vi "AO Regs Group UI.vi"(8 "error in (no error)":errorcluster, 11 "Node Ptr":T2 format="%.0x") -> (0 "error out":errorcluster)   [LabVIEW 2015, in "Modbus Master System Explorer.lvlib"]
uses:
  Modbus Master System Explorer.lvlib
  <vilib>/NI Veristand/Custom Device API/Custom Device Item Ref.ctl
  SubVIs/Conflict Table.ctl
  SubVIs/Modbus Type.ctl
  Shared/Controls/Data Model/Mapping.ctl
  Shared/Controls/Data Model/DataType.ctl
  <vilib>/NI VeriStand/Custom Device API/Custom Device API.lvlib
  <vilib>/NI VeriStand/Custom Device Tools/Custom Device Utility Library/Custom Device Utility Library.lvlib
  Shared/Modbus Master Shared.lvlib
panel:
  in  "Add One":bool
  in  "Bulk Add":bool
  out "Conflicting Holding Register Mappings":T1
  in  "Header":cluster{"Section Name":string}={"Section Name"="Discrete Input Settings"}
  in  "Description":string
  in  "Name":string
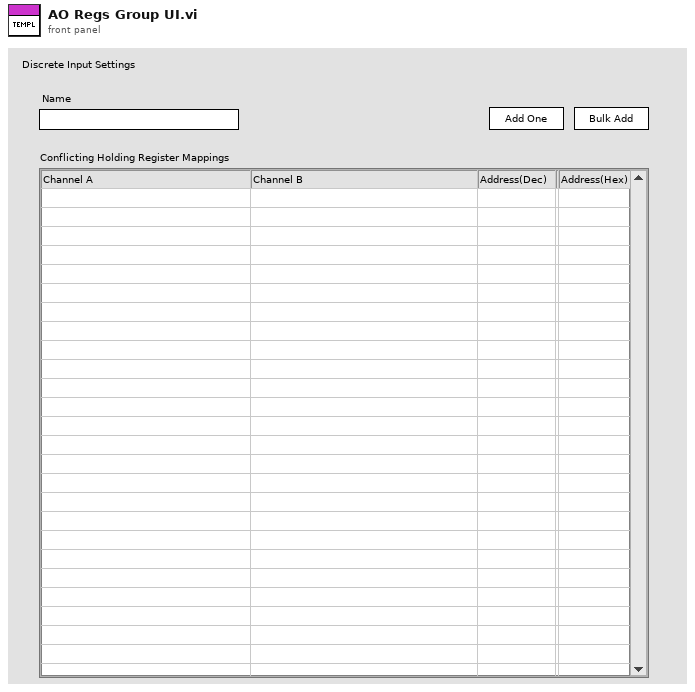
[diagram p1: front panel]
types:
  T1 = typedef "Conflict Table.ctl" = i32
  T2 = typedef "Custom Device API.lvlib/Custom Device Item Ref.ctl" = u64
  T3 = typedef "Custom Device API.lvlib/Custom Device Item Info.ctl" = cluster{"Name":string, "Is Channel":bool, "GUID":string, "Is Waveform":bool}
  T4 = cluster{"Name":string, "Name":string, "Mapping":u16}[]
  T5 = typedef "Modbus Master Shared.lvlib/Modbus Type.ctl" = enum16{"Coil", "Discrete Input", "Holding Register", "Input Register"}
  T6 = typedef "Modbus Master Shared.lvlib/Mapping.ctl" = cluster{"DataType":T7, "Starting Address":u16, "Sub-Index (Bool)":u16, "VS Reference":T2}
  T7 = typedef "Modbus Master Shared.lvlib/DataType.ctl" = enum16{"Double", "Single", "I64", "I32", "I16", "I8", "U64", "U32", "U16", "U8", "Boolean"}
  T8 = typedef "Custom Device API.lvlib/Custom Device Commands.ctl" = enum16{"Default", "Item renamed", "Shutdown", "Dynamic button pressed"}
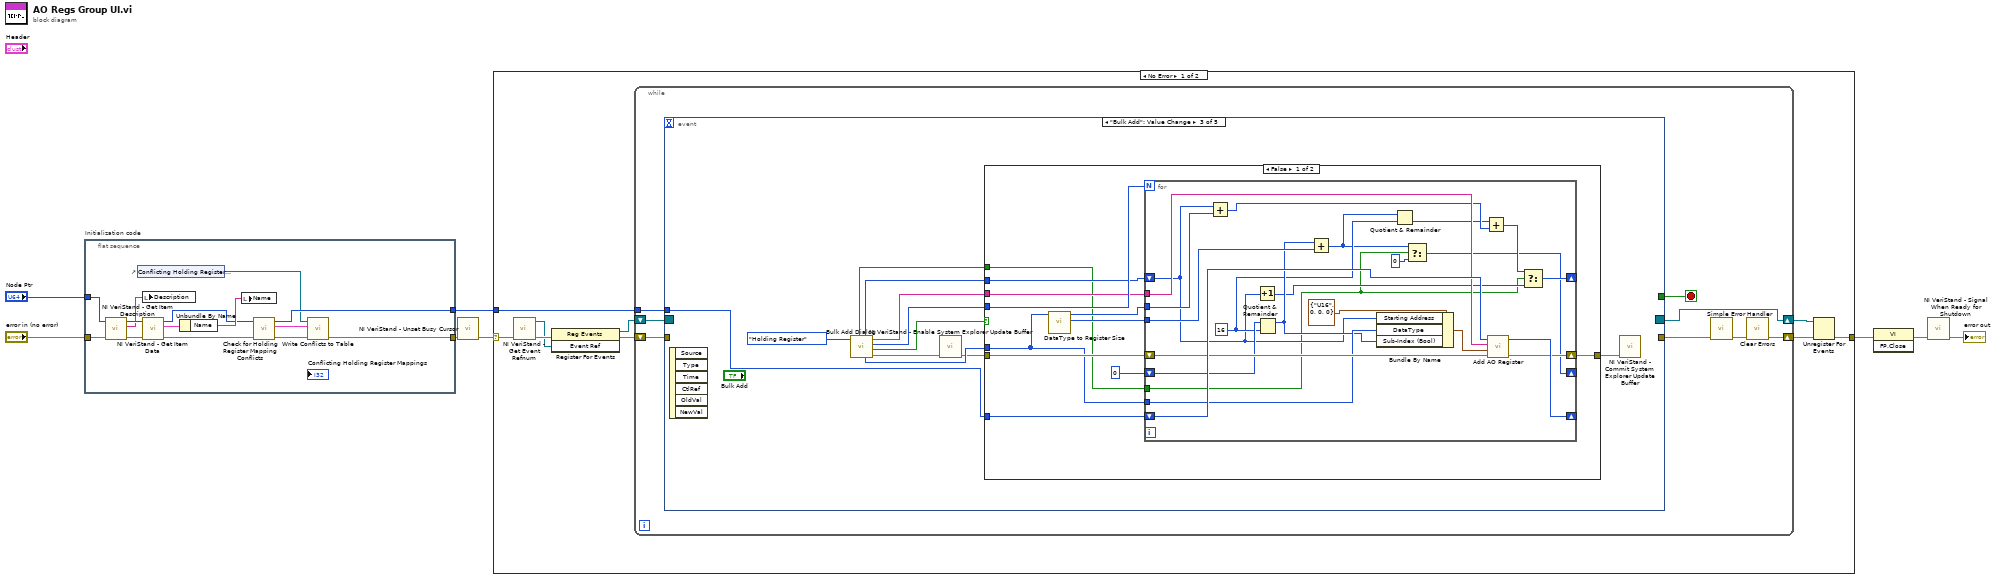
[diagram p0: block diagram]
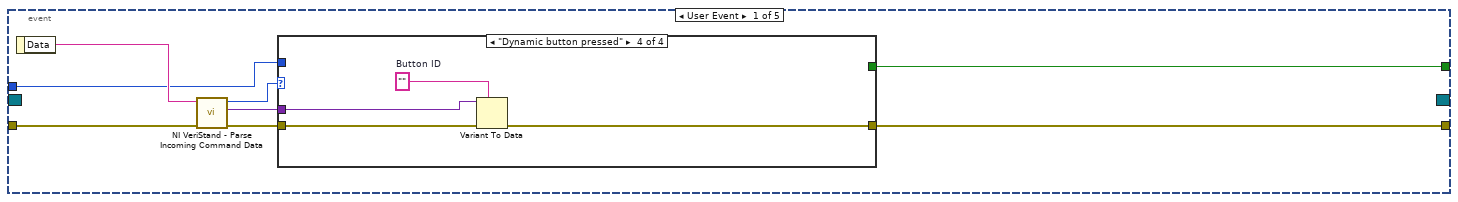
[diagram p2: hidden frame]
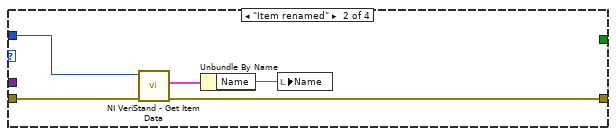
[diagram p4: hidden frame]
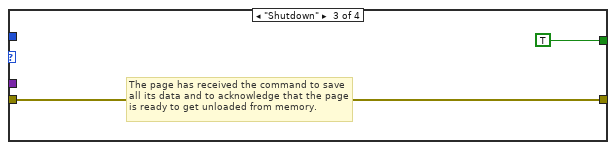
[diagram p5: hidden frame]
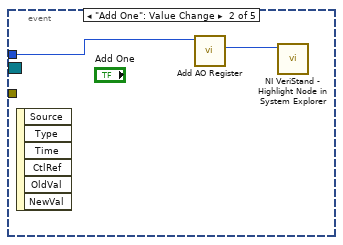
[diagram p6: hidden frame]
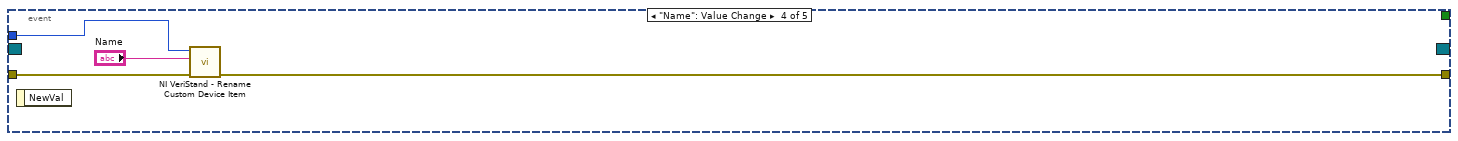
[diagram p8: hidden frame]
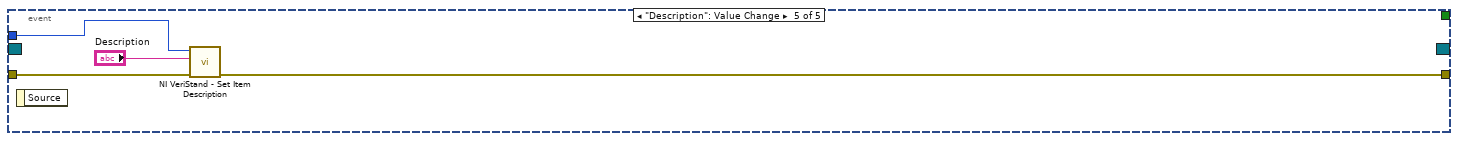
[diagram p9: hidden frame]
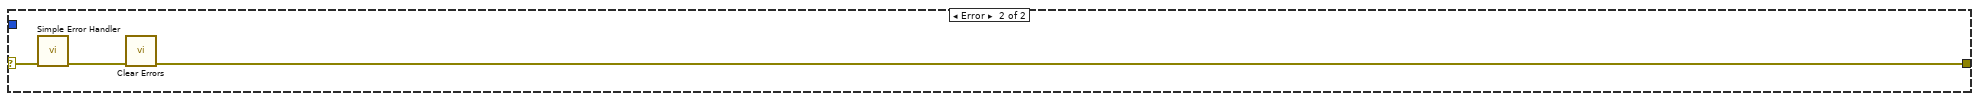
[diagram p10: hidden frame]
diagram:
  n1 = flat-sequence "Initialization code" {
    tunnel: "error in (no error)" -> [w21]
    tunnel: "Node Ptr" -> [w20]
    tunnel: [w12] -> w4
    tunnel: [w14] -> w1
    frame #0 {
      n2 = call <vilib>:"NI VeriStand - Get Item Description.vi"("error in (no error)"=w21, "Item Ref in"=w20) -> ("error out"=w18:errorcluster, "Description"=w19:string, "Item Ref out"=w22:T2)  [unwired: 7 out]
      n3 = control-ref of="Conflicting Holding Register Mappings"() -> (w9:refnum<vi>)
      n4 = local write "Description"(w19) -> ()
      n5 = call <vilib>:"NI VeriStand - Get Item Data.vi"("error in (no error)"=w18, "Item Ref in"=w22) -> ("error out"=w13:errorcluster, "Item Info"=w17:T3, "Item Ref out"=w15:T2)  [unwired: 7 out]
      n6 = Unbundle By Name(w17) -> ("Name"=w16:string)
      n7 = local write "Name"(w16) -> ()
      n8 = call "Check for Holding Register Mapping Conflicts.vi"("error in (no error)"=w13, "Group Ref in"=w15) -> ("error out"=w11:errorcluster, "Conflicts"=w10:T4, "Coil Group Ref out"=w14:T2)  [unwired: 6 in, 1 out]
      n9 = call "Write Conflicts to Table.vi"("error in (no error)"=w11, "Conflicts"=w10, "MC Listbox Ref"=w9) -> ("error out"=w12:errorcluster)  [unwired: 8 in]
    }
  }
  n10 = call <vilib>:"NI VeriStand - Unset Busy Cursor.vi"("error in (no error)"=w4) -> ("error out"=w3:errorcluster)  [unwired: 10 out]
  n11 = case shown="No Error" w3 {
    selector: w3 -> [w23 w118]
    tunnel: [w28 w116] -> w8
    tunnel: w1 -> [w24 _]
    frame No Error {
      n12 = call <vilib>:"NI VeriStand - Get Event Refnum.vi"("error in (no error)"=w23) -> ("error out"=w31:errorcluster, "Event Ref"=w27:refnum<user-event>)  [unwired: 9 out]
      n13 = register-events(error in=w31, w27) -> (reference out=w25:refnum<event-registration>, error out=w26:errorcluster)  [unwired: 1 in]
      n14 = while {
        tunnel: w24 -> [w35]
        shift-right: [w32] -> w29
        shift-left: w26 -> [w38]
        shift-right: [w39] -> w30
        shift-left: w25 -> [w37]
        stop <- w36 stop-if-true
        n15 = event shown="[2] \"Bulk Add\": Value Change" {
          selector: w37 -> [_ _ _ _ _]
          dyn-events: [_ _ _ _ _] -> w39
          timeout: _ -> [_ _ _ _ _]
          tunnel: w38 -> [w47 _ _ w111 w114]
          tunnel: [w43 _ _ _ _] -> w36
          tunnel: [w42 _ _ w110 w113] -> w34
          tunnel: w35 -> [w41 w60 w62 w109 w115]
          event User Event {
            n16 = event-data() -> ("Data"=w46:string)  [unwired: 1 out]
            n17 = call <vilib>:"NI VeriStand - Parse Incoming Command Data.vi"("error in (no error)"=w47, "Incoming data"=w46) -> ("error out"=w45:errorcluster, "Outgoing data"=w40:variant, "Action"=w44:T8)  [unwired: 7 out]
            n18 = case shown="\"Dynamic button pressed\"" w44 {
              tunnel: w45 -> [w48 w53 w54 w59]
              tunnel: [_ _ TRUE _] -> w43
              tunnel: [w48 w50 w54 w56] -> w42
              tunnel: w41 -> [_ w52 _ _]
              tunnel: w40 -> [_ _ _ w58]
              frame "Default", Default {
              }
              frame "Item renamed" {
                n19 = call <vilib>:"NI VeriStand - Get Item Data.vi"("error in (no error)"=w53, "Item Ref in"=w52) -> ("error out"=w50:errorcluster, "Item Info"=w51:T3)  [unwired: 8 out]
                n20 = Unbundle By Name(w51) -> ("Name"=w49:string)
                n21 = local write "Name"(w49) -> ()
              }
              frame "Shutdown" {
                # "The page has received the command to save all its data and to acknowledge that the page is ready to get unloaded from memory."
              }
              frame "Dynamic button pressed" {
                w57 = ""  # Button ID
                n22 = Variant To Data(error in=w59, type=w57, Variant=w58) -> (error out=w56:errorcluster)  [unwired: 1 out]
              }
            }
          }
          event "Add One": Value Change {
            n23 = event-data() -> ()  [unwired: 7 out]
            n24 = call "Add AO Register.vi"("Node Ref In"=w60) -> ("Channel Ref out"=w61:T2)  [unwired: 8 in, 2 out]
            n25 = call <vilib>:"NI VeriStand - Highlight Node in System Explorer.vi"("Item Ref in"=w61) -> ()  [unwired: 9 in, 2 out]
          }
          event "Bulk Add": Value Change {
            n26 = event-data() -> ()  [unwired: 7 out]
            n27 = call "Bulk Add Dialog.vi"("Type"=Modbus_Type."Holding Register") -> ("error out"=w66:errorcluster, "Cancelled?"=w69:bool, "Quantity Out"=w70:u16, "Root Name Out"=w71:string, "DataType Out"=w68:T7, "Starting Address Out"=w72:u16, "Pack Values? Out"=w67:bool)  [unwired: 4 in]
            n28 = call <vilib>:"NI VeriStand - Enable System Explorer Update Buffer.vi"("error in (no error)"=w66) -> ("error out"=w65:errorcluster)  [unwired: 10 in]
            n29 = case shown="False" w69 {
              tunnel: w62 -> [w76 _]
              tunnel: w70 -> [w83 _]
              tunnel: w65 -> [w77 w107]
              tunnel: w71 -> [w82 _]
              tunnel: w72 -> [w81 _]
              tunnel: w68 -> [w75 _]
              tunnel: w67 -> [w74 _]
              tunnel: [w73 w107] -> w64
              frame False {
                n30 = call "DataType to Register Size.vi"("DataType"=w75) -> ("bits"=w78:i32, "bytes"=w80:i32)  [unwired: 9 in]
                n31 = for {
                  N: w83 -> [_]
                  shift-right: [w104] -> _
                  shift-left: w76 -> [w106]
                  shift-right: [w102] -> w73
                  shift-left: w77 -> [w105]
                  tunnel: w82 -> [w103]
                  shift-right: [w89] -> _
                  shift-left: w81 -> [w91]
                  tunnel: w75 -> [w100]
                  tunnel: w80 -> [w99]
                  shift-right: [w86] -> _
                  shift-left: 0 ("Sub-Index (Bool)") -> [w97]
                  tunnel: w78 -> [w98]
                  tunnel: w74 -> [w88]
                  w94 = 16 ("y")
                  n32 = Add(x=w91, y=w99) -> (x+y=w95:i32)
                  n33 = Increment(x=w91) -> (x+1=w92:i32)
                  n34 = Quotient & Remainder(x=w97, y=w94) -> (x-y*floor(x/y)=w96:i32)  [unwired: 1 out]
                  n35 = Add(x=w96, y=w98) -> (x+y=w87:i32)
                  n36 = Bundle By Name(cluster=T6 {"DataType"=enum."U16", "Starting Address"=0, "Sub-Index (Bool)"=0, "VS Reference"=0} ("Mapping"), "Starting Address"=w91, "DataType"=w100, "Sub-Index (Bool)"=w96) -> (w84:T6)
                  n37 = Quotient & Remainder(x=w87, y=w94) -> (floor(x/y)=w93:i32)  [unwired: 1 out]
                  n38 = Select(t=w87, s=w88, f=0 ("t")) -> (s? t:f=w86:i32)
                  n39 = Add(x=w93, y=w95) -> (x+y=w90:i32)
                  n40 = call "Add AO Register.vi"("error in (no error)"=w105, "Mapping"=w84, "Label"=w103, "Node Ref In"=w106) -> ("error out"=w102:errorcluster, "Node Ref out"=w104:T2)  [unwired: 5 in, 1 out]
                  n41 = Select(t=w90, s=w88, f=w92) -> (s? t:f=w89:i32)
                }
              }
              frame True {
              }
            }
            n42 = call <vilib>:"NI VeriStand - Commit System Explorer Update Buffer.vi"("error in (no error)"=w64) -> ()  [unwired: 10 in, 1 out]
          }
          event "Name": Value Change {
            n43 = event-data() -> ()  [unwired: 2 out]
            n44 = call <vilib>:"NI VeriStand - Rename Custom Device Item.vi"("error in (no error)"=w111, "New Name"="Name", "Item Ref in"=w109) -> ("error out"=w110:errorcluster)  [unwired: 1 in, 7 out]
          }
          event "Description": Value Change {
            n45 = event-data() -> ()  [unwired: 2 out]
            n46 = call <vilib>:"NI VeriStand - Set Item Description.vi"("error in (no error)"=w114, "Description"="Description", "Item Ref in"=w115) -> ("error out"=w113:errorcluster)  [unwired: 8 out]
          }
        }
        n47 = call <vilib>:"Simple Error Handler.vi"("error in (no error)"=w34) -> ("error out"=w33:errorcluster)  [unwired: 1 in, 7 out]
        n48 = call <vilib>:"Clear Errors.vi"("error in (no error)"=w33) -> ("error out"=w32:errorcluster)  [unwired: 1 in, 5 out]
      }
      n49 = Unregister For Events(event registration refnum=w30, error in=w29) -> (error out=w28:errorcluster)
    }
    frame Error {
      n50 = call <vilib>:"Simple Error Handler.vi"("error in (no error)"=w118) -> ("error out"=w117:errorcluster)  [unwired: 1 in, 7 out]
      n51 = call <vilib>:"Clear Errors.vi"("error in (no error)"=w117) -> ("error out"=w116:errorcluster)  [unwired: 1 in, 5 out]
    }
  }
  n52 = invoke class="VI" method="FP.Close"(error in=w8) -> (error out=w7:errorcluster)  [unwired: 2 in, 2 out]
  n53 = call <vilib>:"NI VeriStand - Signal When Ready for Shutdown.vi"("error in (no error)"=w7) -> ("error out"=→"error out":errorcluster)  [unwired: 10 out]
